vi "PASS-FAIL (SubVI).vi"(0 "PASS Button":bool, 2 "FAIL Button":bool, 5 "Clear PASS/FAIL Selection":bool) -> (14 "PASS/FAIL Latch":bool, 15 "PASS/FAIL String":string, 16 "PASS Pulse":bool, 17 "FAIL Pulse":bool, 19 "PASS/FAIL Pulse":bool)   [LabVIEW 2009]
panel:
  # "PASS-FAIL SubVI\nCreated by Blake Otting\n4/14/2010"
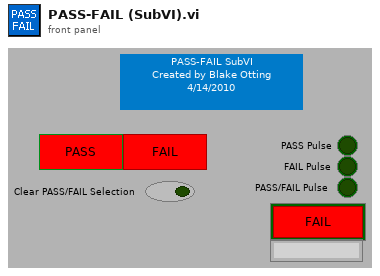
[diagram p1: front panel]
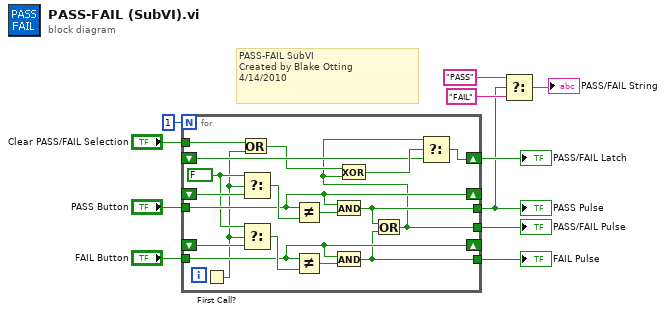
[diagram p0: block diagram]
diagram:
  # "PASS-FAIL SubVI\nCreated by Blake Otting\n4/14/2010"
  n1 = for {
    N: 1 -> [_]
    tunnel: "PASS Button" -> [w26]
    tunnel: "FAIL Button" -> [w22]
    shift-right: [w26] -> _
    shift-left: _ -> [w29]
    tunnel: [w20] -> w1
    tunnel: [w19] -> w10
    shift-right: [w22] -> _
    shift-left: _ -> [w23]
    tunnel: [w12] -> w9
    shift-right: [w17] -> w5
    shift-left: _ -> [w16]
    tunnel: "Clear PASS/FAIL Selection" -> [w14]
    w21 = FALSE ("t")
    n2 = First Call?() -> (First Call?: T/F=w15:bool)
    n3 = Or(x=w14, y=w15) -> (x .or. y?=w13:bool)
    n4 = Select(t=w21, s=w15, f=w29) -> (s? t:f=w28:bool)
    n5 = Select(t=w21, s=w15, f=w23) -> (s? t:f=w25:bool)
    n6 = Not Equal?(x=w26, y=w28) -> (x != y?=w27:bool)
    n7 = Not Equal?(x=w22, y=w25) -> (x != y?=w24:bool)
    n8 = And(x=w26, y=w27) -> (x .and. y?=w20:bool)
    n9 = And(x=w22, y=w24) -> (x .and. y?=w19:bool)
    n10 = Or(x=w20, y=w19) -> (x .or. y?=w12:bool)
    n11 = Exclusive Or(1:w12, 2:w13) -> (0:w18:bool)
    n12 = Select(t=w12, s=w18, f=w16) -> (s? t:f=w17:bool)
  }
  "PASS/FAIL Pulse" <- w9
  "PASS Pulse" <- w1
  "FAIL Pulse" <- w10
  "PASS/FAIL Latch" <- w5
  n13 = Select(t="PASS", s=w1, f="FAIL") -> (s? t:f=→"PASS/FAIL String":string)
